vi "Rig_Control.vi"() -> ()   [LabVIEW 2011]
panel:
  in  "Rig Name":string
  in  "Cluster array":cluster{"Ch Name":string, "Boolean":bool}[](array[cluster])
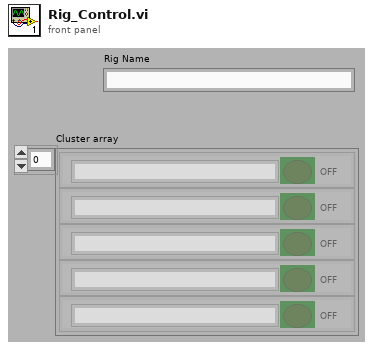
[diagram p1: front panel]
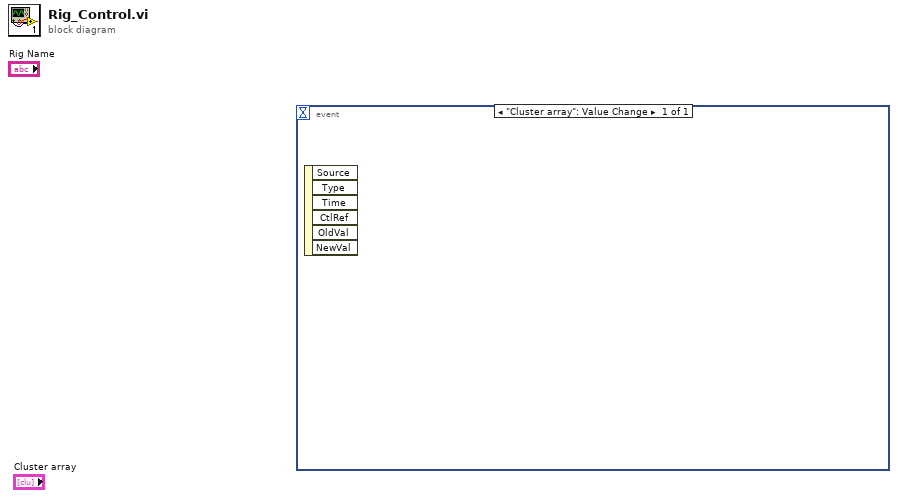
[diagram p0: block diagram]
diagram:
  n1 = event shown="[0] \"Cluster array\": Value Change" {
    selector: _ -> [_]
    dyn-events: _ -> [_]
    timeout: _ -> [_]
    event "Cluster array": Value Change {
      n2 = event-data() -> ()  [unwired: 7 out]
    }
  }
